vi "getMagnet.vi"(6 "Axis":T1=enum."Z", 8 "error in (no error)":errorcluster, 11 "Instrument.Cryostat in":refnum<class "Instrument.Cryostat.lvclass">) -> (0 "error out":errorcluster, 1 "Status":string, 2 "B Field (T)":dbl, 3 "Instrument.Cryostat out":refnum<class "Instrument.Cryostat.lvclass">, 4 "Finished?":bool)   [LabVIEW 2019, in "Instrument.Cryostat.lvclass"]
uses:
  Instrument.Cryostat.lvclass
  C:/Users/patrick/Documents/GitHub/Instrument-Framework/lvsrc/Instrument/Instrument.lvclass
  Typedefs/Magnet Axis--Enum.ctl
  Typedefs/getMagnet--cluster.ctl
  Typedefs/Cryostat.commands--enum.ctl
  396bafcf-3afa-44ea-bca1-bee317a97b09.vi
  396bafcf-3afa-44ea-bca1-bee317a97b09.vi/60e3f191-daa0-4a27-ba83-e38e8ee253d8.vi
  396bafcf-3afa-44ea-bca1-bee317a97b09.vi/60e3f191-daa0-4a27-ba83-e38e8ee253d8.vi/b0aa3784-f3f6-4ea6-85a1-bb775bb1b375.vi
  396bafcf-3afa-44ea-bca1-bee317a97b09.vi/60e3f191-daa0-4a27-ba83-e38e8ee253d8.vi/9b7ceede-b888-4fee-a67b-9c34e9c43dcf.vi
  Instrument/Protected/Validate API method.vi
  Instrument/Private/Get RC Connection Status.vi
  Instrument/API/Send and Receive.vi
  <vilib>/Utility/Data Type/Get Type Information.vi
  <vilib>/JDP Science/JSONtext/JSON text to Variant.vi
  <vilib>/JDP Science/JSONtext/LVClass Serializer/JSONtext LVClass Serializer.lvclass
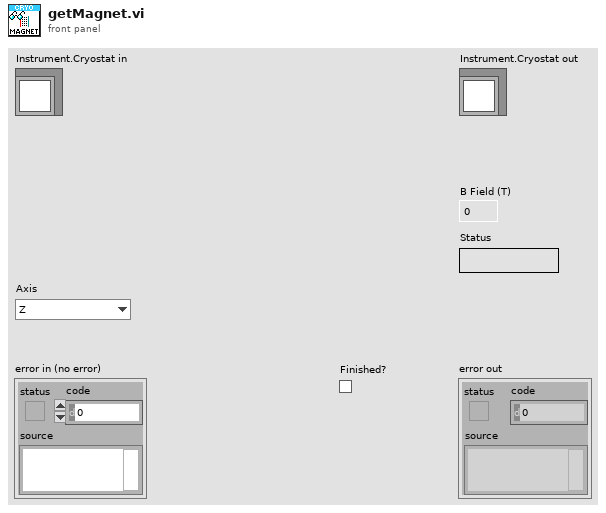
[diagram p1: front panel]
types:
  T1 = typedef "Instrument.Cryostat.lvclass/Magnet Axis--Enum.ctl" = enum16{"X", "Y", "Z"}
  T2 = typedef "Instrument.Cryostat.lvclass/Cryostat.commands--enum.ctl" = enum16{"getLN2Level", "getLHeLevel", "getMagnet", "getMagnetVector", "setMagnet", "setMagnetVector", "getAngle", "setAngle", "getTemperature", "setTemperature", "getHeater", "setHeater", "getChamber", "setChamber", "getPressure"}
  T3 = typedef "Instrument.Cryostat.lvclass/getMagnet--cluster.ctl" = cluster{"field":dbl, "status":string, "finished":bool}
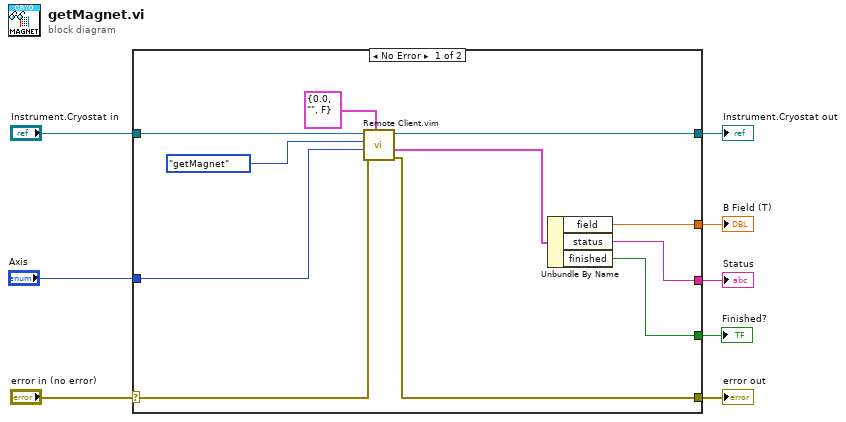
[diagram p0: block diagram]
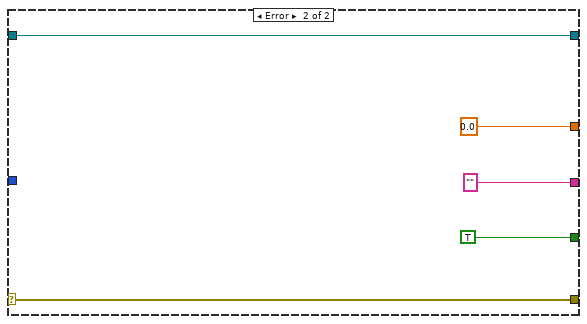
[diagram p2: hidden frame]
diagram:
  n1 = case shown="No Error" "error in (no error)" {
    selector: "error in (no error)" -> [w10 w24]
    tunnel: [w13 w24] -> w7
    tunnel: [w19 w23] -> w5
    tunnel: "Instrument.Cryostat in" -> [w12 w23]
    tunnel: "Axis" -> [w18 _]
    tunnel: [w17 0.0 ("Field (T)")] -> w3
    tunnel: [w16 "" ("Status")] -> w2
    tunnel: [w15 TRUE] -> w1
    frame No Error {
      n2 = call "Remote Client.vim"("Data Out type"=T3 {"field"=0.0, "status"="", "finished"=FALSE} ("getMagnet"), "error in (no error)"=w10, "Data in"=w18, "Command in"=Cryostat.commands--enum."getMagnet" ("commands"), "Instrument in"=w12) -> ("error out"=w13:errorcluster, "Data out"=w14:T3, "Instrument out"=w19:refnum<class "Instrument.Cryostat.lvclass">)  [unwired: 3 in, 1 out]
      n3 = Unbundle By Name(w14) -> ("field"=w17:dbl, "status"=w16:string, "finished"=w15:bool)
    }
    frame Error {
    }
  }
  "error out" <- w7
  "Instrument.Cryostat out" <- w5
  "B Field (T)" <- w3
  "Status" <- w2
  "Finished?" <- w1
